vi "(TestVI)example_scope_while loop.vi"() -> ()   [LabVIEW 2020]
uses:
  Serial/Controls/(Ctrl)Serial_FGV Function.ctl
panel:
  in  "Register":u16[](array[numeric])=[0] format="%.0x"
  out "Scope_Data":i16[][](graph) caption="Data"
  in  "정지":bool
  in  "User Code":u8
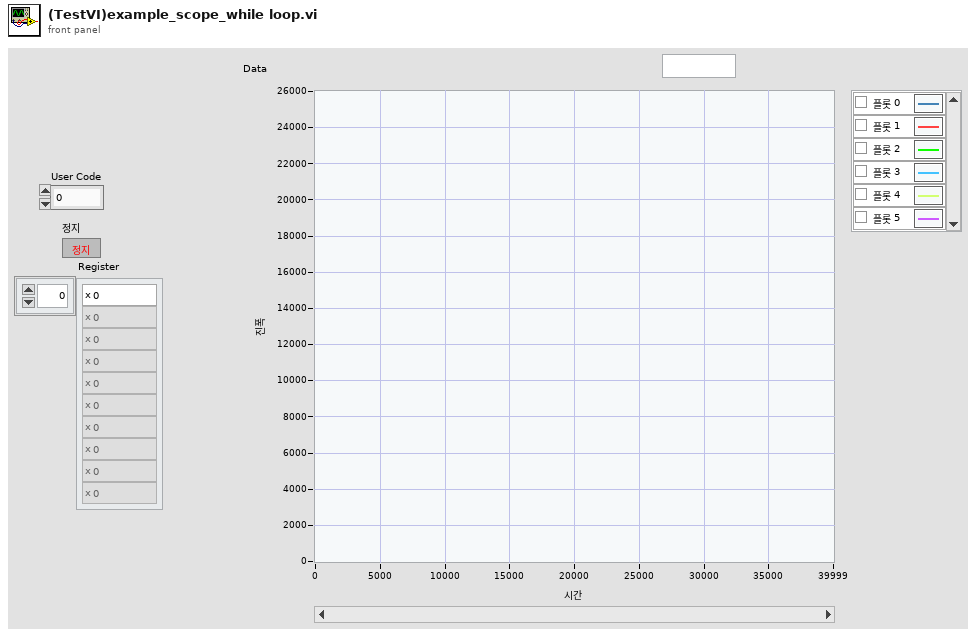
[diagram p1: front panel]
types:
  T1 = typedef "(Ctrl)Serial_FGV Function.ctl" = enum16{"Initialize", "Read", "Read All", "Write", "Flush Buffer", "Get Ref.", "Close"}
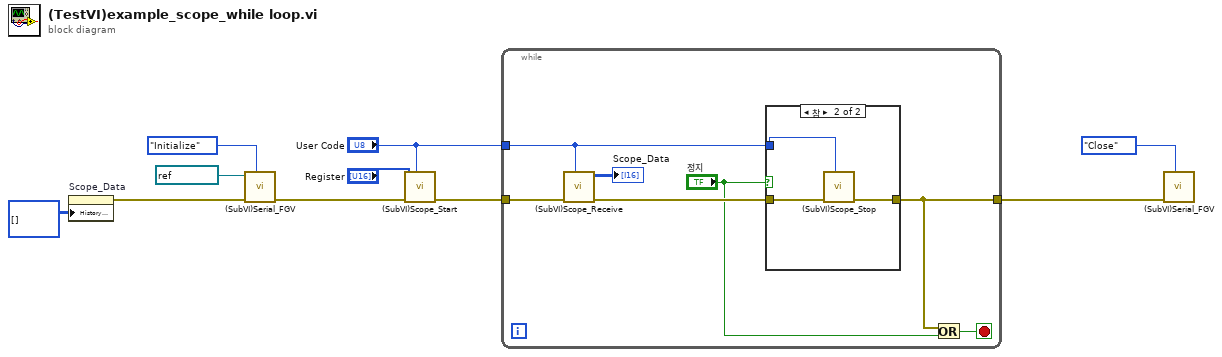
[diagram p0: block diagram]
diagram:
  n1 = property on="Scope_Data" class="WFChart (엄격한)"("History Data"=i32[][] [] ("히스토리 데이터")) -> (error out=w2:errorcluster)  [unwired: 2 in, 1 out]
  n2 = call "(SubVI)Serial_FGV.vi"("Function"=(Ctrl)Serial_FGV_Function."Initialize", "error in (no error)"=w2, "VISA resource name"=refnum<visa-resource-name> "COM3") -> ("error out"=w7:errorcluster)  [unwired: 6 in, 2 out]
  n3 = call "(SubVI)Scope_Start.vi"("Mode"="User Code", "error in (no error)"=w7, "Recording Time"="Register") -> ("error out"=w6:errorcluster)  [unwired: 8 in]
  n4 = while {
    tunnel: "User Code" -> [w15]
    tunnel: w6 -> [w17]
    tunnel: [w11] -> w5
    stop <- w12 stop-if-true
    n5 = call "(SubVI)Scope_Receive.vi"("User Code"=w15, "error in (no error)"=w17) -> ("error out"=w16:errorcluster, "Data"=→"Scope_Data":i16[][])  [unwired: 7 in, 1 out]
    n6 = case shown="참" "정지" {
      tunnel: w16 -> [w18 w21]
      tunnel: [w18 w20] -> w11
      tunnel: w15 -> [_ w19]
      frame False {
      }
      frame True {
        n7 = call "(SubVI)Scope_Stop.vi"(7:w19, "error in (no error)"=w21) -> ("error out"=w20:errorcluster)  [unwired: 9 in]
      }
    }
    n8 = Or(x=w11, y="정지") -> (x .or. y?=w12:bool)
  }
  n9 = call "(SubVI)Serial_FGV.vi"("Function"=(Ctrl)Serial_FGV_Function."Close", "error in (no error)"=w5) -> ()  [unwired: 7 in, 3 out]
